vi "Norm_vector_3x1 (SubVI).vi"(11 "Vector":sgl[](array[numeric])) -> (3 "Norm":sgl)   [LabVIEW 2017]
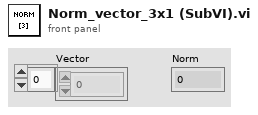
[diagram p1: front panel]
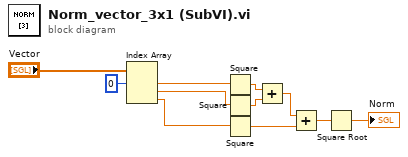
[diagram p0: block diagram]
diagram:
  n1 = Index Array(array="Vector", index #1=0 ("index")) -> (element #1=w3:sgl, element #2=w4:sgl, element #3=w5:sgl)  [unwired: 2 in]
  n2 = Square(x=w3) -> (x^2=w6:sgl)
  n3 = Square(x=w4) -> (x^2=w7:sgl)
  n4 = Square(x=w5) -> (x^2=w9:sgl)
  n5 = Add(x=w6, y=w7) -> (x+y=w8:sgl)
  n6 = Add(x=w8, y=w9) -> (x+y=w10:sgl)
  n7 = Square Root(x=w10) -> (sqrt(x)=→"Norm":sgl)
